vi "DAC Run.vi"(8 "error in":errorcluster, 11 "DAC Shunt dU in":refnum<class "DAC Shunt dU.lvclass">) -> (0 "error out":errorcluster, 3 "DAC Shunt dU out":refnum<class "DAC Shunt dU.lvclass">)   [LabVIEW 2019, in "DAC.lvlib" / "DAC Shunt dU.lvclass"]
uses:
  DAC Shunt dU.lvclass
  C:/Users/wg/Documents/LV_Projects/TestStand/App/DAC/DAC.lvclass
  DAC.lvclass/DAC.ctl
  Results/LNG Boiling Results/LNG Boiling Results.lvclass
  Results/Results Method.ctl
  DAC Shunt dU.lvclass/DAC Shunt dU.ctl
  Results/LNG Boiling Results/LNG Boiling Results.lvclass/LNG Boiling Results.ctl
  <vilib>/DAQmx/read.llb/DAQmx Read (Analog DBL 1Chan 1Samp).vi
  <vilib>/DAQmx/miscellaneous.llb/DAQmx Fill In Error Info.vi
  DAC.lvclass
  Results/Results.lvlib
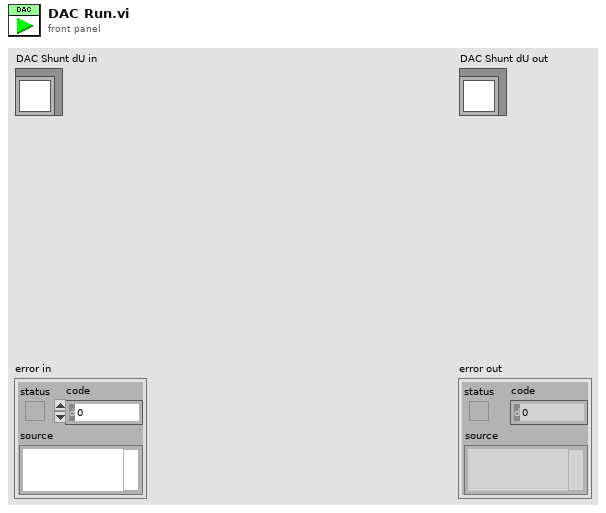
[diagram p1: front panel]
types:
  T1 = typedef "Results.lvlib/Results Method.ctl" = enum16{"Get", "Set"}
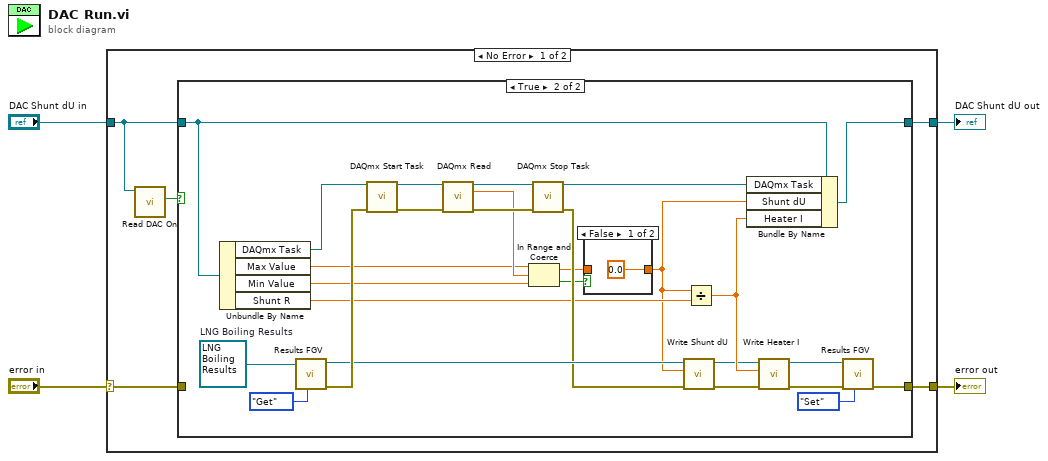
[diagram p0: block diagram]
diagram:
  n1 = case shown="No Error" "error in" {
    selector: "error in" -> [w7 w42]
    tunnel: [w6 w42] -> w2
    tunnel: [w8 w41] -> w1
    tunnel: "DAC Shunt dU in" -> [w5 w41]
    frame No Error {
      n2 = call "Read DAC On.vi"("DAC in"=w5) -> ("DAC On"=w9:bool)  [unwired: 8 in, 2 out]
      n3 = case shown="True" w9 {
        tunnel: w5 -> [w11 w34]
        tunnel: [w11 w25] -> w8
        tunnel: w7 -> [w10 _]
        tunnel: [w10 w24] -> w6
        frame False {
        }
        frame True {
          w33 = refnum<class "LNG Boiling Results.lvclass"> refnum  # LNG Boiling Results
          n4 = Unbundle By Name(w34) -> ("DAQmx Task"=w38:refnum<k21>, "Max Value"=w15:dbl, "Min Value"=w16:dbl, "Shunt R"=w17:dbl)
          n5 = call-dynamic "Results FGV.vi"("Method"=Results_Method."Get", "LNG Boiling Results in"=w33) -> ("error out"=w30:errorcluster, "LNG Boiling Results out"=w22:refnum<class "LNG Boiling Results.lvclass">)  [unwired: 8 in]
          n6 = call <vilib>:"DAQmx Start Task.vi"("task/channels in"=w38, "error in"=w30) -> ("task out"=w37:refnum<k21>, "error out"=w36:errorcluster)  [unwired: 12 in]
          n7 = call-poly <vilib>:"DAQmx Read.vi"("task/channels in"=w37, "error in"=w36) -> ("task out"=w26:refnum<k21>, "data"=w18:dbl, "error out"=w35:errorcluster)  [unwired: 11 in]
          n8 = In Range and Coerce(upper limit=w15, x=w18, lower limit=w16) -> (coerced(x)=w13:dbl, In Range?=w14:bool)
          n9 = call <vilib>:"DAQmx Stop Task.vi"("task/channels in"=w26, "error in"=w35) -> ("task out"=w27:refnum<k21>, "error out"=w21:errorcluster)  [unwired: 12 in]
          n10 = case shown="False" w14 {
            tunnel: w13 -> [_ w40]
            tunnel: [0.0 ("Max Value") w40] -> w12
            frame False {
            }
            frame True {
            }
          }
          n11 = call "Write Shunt dU.vi"("error in (no error)"=w21, "Shunt dU"=w12, "LNG Boiling Results in"=w22) -> ("error out"=w19:errorcluster, "LNG Boiling Results out"=w20:refnum<class "LNG Boiling Results.lvclass">)  [unwired: 7 in]
          n12 = Divide(x=w12, y=w17) -> (x/y=w23:dbl)
          n13 = Bundle By Name(cluster=w34, "DAQmx Task"=w27, "Shunt dU"=w12, "Heater I"=w23) -> (w25:refnum<class "DAC Shunt dU.lvclass">)
          n14 = call "Write Heater I.vi"("error in (no error)"=w19, "Heater I"=w23, "LNG Boiling Results in"=w20) -> ("error out"=w28:errorcluster, "LNG Boiling Results out"=w29:refnum<class "LNG Boiling Results.lvclass">)  [unwired: 7 in]
          n15 = call-dynamic "Results FGV.vi"("Method"=Results_Method."Set", "error in"=w28, "LNG Boiling Results in"=w29) -> ("error out"=w24:errorcluster)  [unwired: 7 in, 1 out]
        }
      }
    }
    frame Error {
    }
  }
  "error out" <- w2
  "DAC Shunt dU out" <- w1
